vi "ConvertTo(MoveAllAbsolute).vi"(8 "error in":errorcluster, 9 "Message Payload":variant) -> (0 "error out":errorcluster, 1 "Message Payload Move":T1)   [LabVIEW 2017]
doc: "Convert variant to DBL scalar\n\nBolder Software LLC"
uses:
  MoveAllAbsolute.ctl
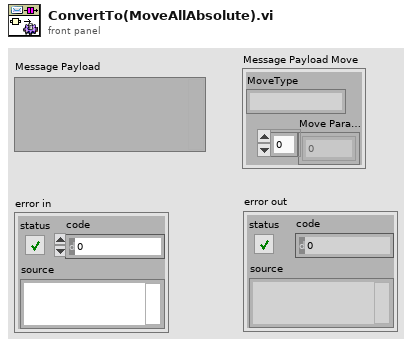
[diagram p1: front panel]
types:
  T1 = typedef "MoveAllAbsolute.ctl" = cluster{"MoveType":string, "Move Params":dbl[]}
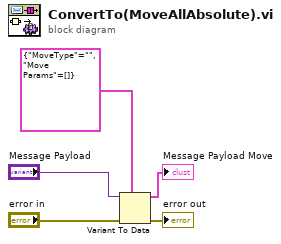
[diagram p0: block diagram]
diagram:
  n1 = Variant To Data(error in="error in", type=T1 {"MoveType"="", "Move Params"=[]}, Variant="Message Payload") -> (data=→"Message Payload Move":T1, error out=→"error out":errorcluster)
